vi "WB_import_separate_sub.vi"(0 "weights&Biases_cvs_file path":path=path "C:/Users/박원일/NEPL Dropbox/연구실 공용/뉴로모픽 과제/weights/weights_f_93.csv", 2 "format (%.3f)":string="%.3f") -> (3 "max value":dbl, 4 "min value":dbl, 5 "Weights & Biases":dbl[][](array[numeric]), 6 "Weights":dbl[][](array[numeric]), 7 "Biases":dbl[](array[numeric]), 8 "No.Input":i32, 9 "No.Output":i32)   [LabVIEW 2021]
uses:
  <vilib>/Utility/file.llb/Read Delimited Spreadsheet (DBL).vi
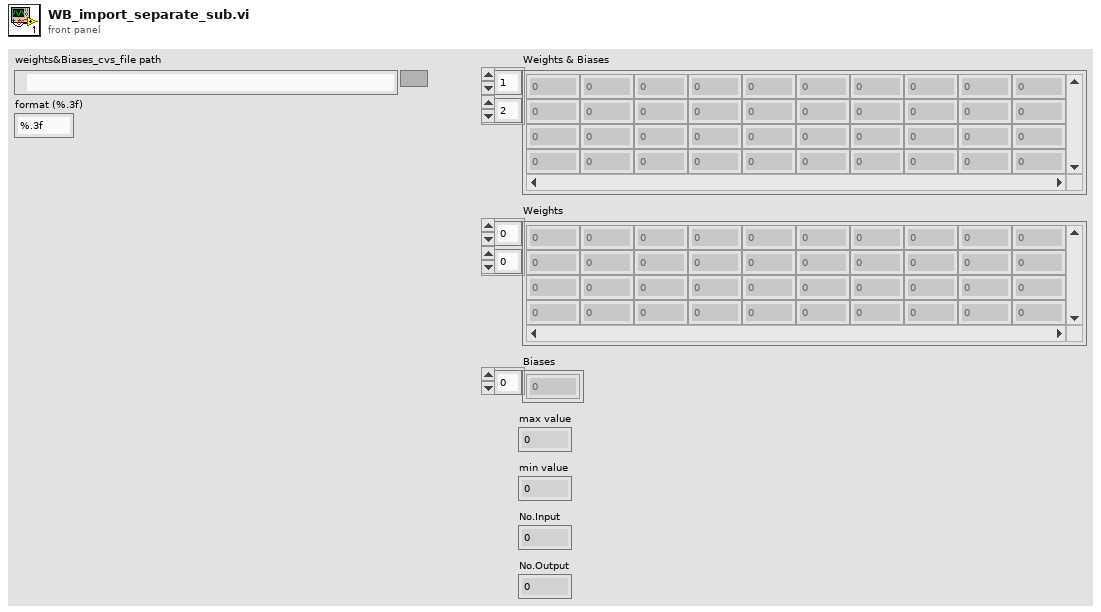
[diagram p1: front panel]
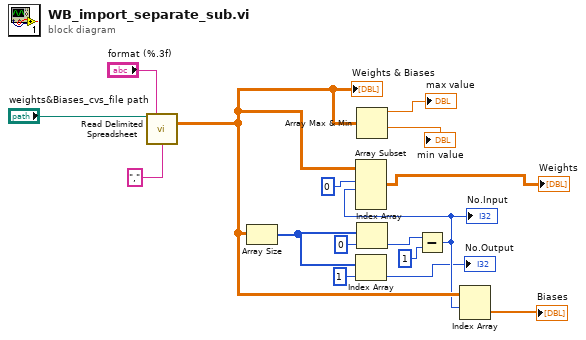
[diagram p0: block diagram]
diagram:
  n1 = call-poly <vilib>:"Read Delimited Spreadsheet.vi"("file path (dialog if empty)"="weights&Biases_cvs_file path", "format (%.3f)"="format (%.3f)", "delimiter (\\t)"="," ("delimiter (\\t)")) -> ("all rows"=w10:dbl[][])  [unwired: 7 in, 5 out]
  "Weights & Biases" <- w10
  n2 = Array Size(array=w10) -> (size(s)=w8:i32[])
  n3 = Index Array(array=w8, index=1 ("인덱스")) -> (element=→"No.Output":i32)
  n4 = Array Max & Min(array=w10) -> (max value=→"max value":dbl, min value=→"min value":dbl)  [unwired: 2 out]
  n5 = Index Array(array=w8, index=0 ("인덱스")) -> (element=w6:i32)
  n6 = Subtract(x=w6, y=1) -> (x-y=w4:i32)
  "No.Input" <- w4
  n7 = Array Subset(array=w10, index (row)=0 ("인덱스"), length (row)=w4) -> (→"Weights":dbl[][])  [unwired: 2 in]
  n8 = Index Array(array=w10, index (row)=w4) -> (element=→"Biases":dbl[])  [unwired: 1 in]
